vi "LED Spike Wrapper.vi"(1 "Camera LED ON/OFF":bool, 2 "Mode":enum8{"Start", "Run", "Finish"}(ring)) -> ()   [LabVIEW 2014]
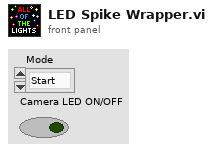
[diagram p1: front panel]
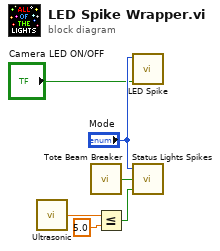
[diagram p0: block diagram]
diagram:
  n1 = call "Ultrasonic.vi"() -> ("Distance"=w5:dbl)  [unwired: 1 in]
  n2 = call "Tote Beam Breaker.vi"() -> ("Boolean"=w6:bool)  [unwired: 1 in]
  n3 = Less Or Equal?(x=w5, y=5.0) -> (x <= y?=w3:bool)
  n4 = call "LED Spike.vi"("ON/OFF"="Camera LED ON/OFF", "Mode"="Mode") -> ()  [unwired: 10 in]
  n5 = call "Status Lights Spikes.vi"("Light  2"=w3, "Light 1"=w6, "Mode"="Mode") -> ()  [unwired: 1 in]
